vi "set_config_cluster.vi"(8 "error in (no error)":errorcluster, 10 "config cluster variant":variant, 11 "FPGAWrapperRK120511Fiber_Spiral in":refnum<class "FPGAWrapperRK110512Fiber_Spiral.lvclass">) -> (0 "error out":errorcluster, 3 "FPGAWrapperRK120511Fiber_Spiral out":refnum<class "FPGAWrapperRK110512Fiber_Spiral.lvclass">)   [LabVIEW 2010, in "FPGAWrapperRK110512Fiber_Spiral.lvclass"]
uses:
  FPGAWrapperRK110512Fiber_Spiral.lvclass
  FPGAWrapperRK110512Fiber_Spiral.lvclass/FPGAWrapperRK110512Fiber_Spiral.ctl
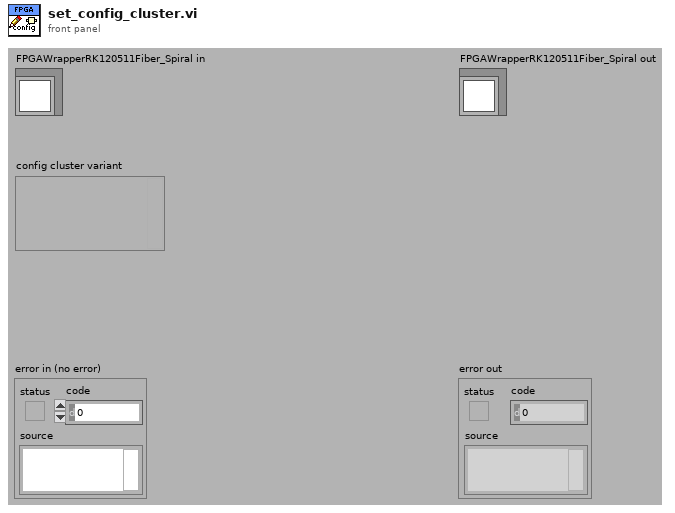
[diagram p1: front panel]
types:
  T1 = typedef "FPGAWrapperRK110512Fiber_Spiral.lvclass/config_data_cluster.ctl" = cluster{"Hifo box version":i16, "ADC clock phase":u8, "Enable ADC clock":bool, "FPGA Clock":u32}
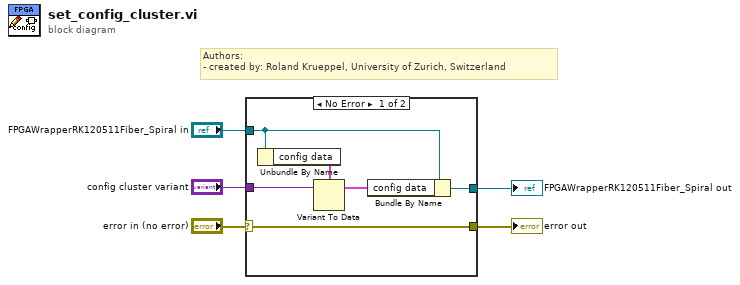
[diagram p0: block diagram]
diagram:
  # "Authors: \n- created by: Roland Krueppel, University of Zurich, Switzerland"
  n1 = case shown="No Error" "error in (no error)" {
    selector: "error in (no error)" -> [w6 w13]
    tunnel: "FPGAWrapperRK120511Fiber_Spiral in" -> [w9 w12]
    tunnel: "config cluster variant" -> [w11 _]
    tunnel: [w7 w12] -> w2
    tunnel: [w6 w13] -> w1
    frame No Error {
      n2 = Unbundle By Name(w9) -> ("config data"=w8:T1)
      n3 = Variant To Data(Variant=w11, type=w8) -> (data=w10:T1)  [unwired: 1 in, 1 out]
      n4 = Bundle By Name(cluster=w9, "config data"=w10) -> (w7:refnum<class "FPGAWrapperRK110512Fiber_Spiral.lvclass">)
    }
    frame Error {
    }
  }
  "error out" <- w1
  "FPGAWrapperRK120511Fiber_Spiral out" <- w2
